vi "SignalSenderLoop.TestLauncher.vi"() -> ()   [LabVIEW 2020, in "ECU_Diagnose.lvlib" / "SignalSenderLoop.lvclass"]
doc: "JKI State Machine Objects (SMO) 1.0.0.5\nJKI - JKI\nCopyright (c) 2016, JKI"
uses:
  SignalSenderLoop.lvclass
  Typedefs/Data.ctl
  Typedefs/PublicEvents--Cluster.ctl
  Typedefs/SetpointChanged--EventData--Cluster.ctl
  <vilib>/JKI/JKI SMO/SMO/Typedefs/Public Events.ctl
  <vilib>/JKI/JKI SMO/SMO/Typedefs/SMOState --Enum.ctl
  <vilib>/JKI/JKI SMO/SMO/Typedefs/Reserve State--Enum.ctl
  <vilib>/JKI/JKI SMO/SMO/SMO.lvclass
  C:/Program Files (x86)/National Instruments/LabVIEW 2020/vi.lib/JKI/JKI SMO/SMO/SMO.lvclass
panel:
  out "SMOArry":refnum<class "SignalSenderLoop.lvclass">[](array[class])
  out "EventHandl(订阅事件用)":refnum<event-registration>[](array[refnum])
  in  "SignalsSet 2":dbl[](array[numeric])=[0.0]
  out "元素":refnum<class "SignalSenderLoop.lvclass">
  in  "SignalsSet":dbl[](array[numeric])=[60.0, 1.0]
  out "Value 3":T1
  out "Value 2":T1
  out "数组":errorcluster[](array[cluster])
  in  "Stop":bool
  # "ECU Signals Sender Test Launcher"
  # "数组为空，不发送任何帧，即停止发送"
  # "数组为空，不发送任何帧，即停止发送"
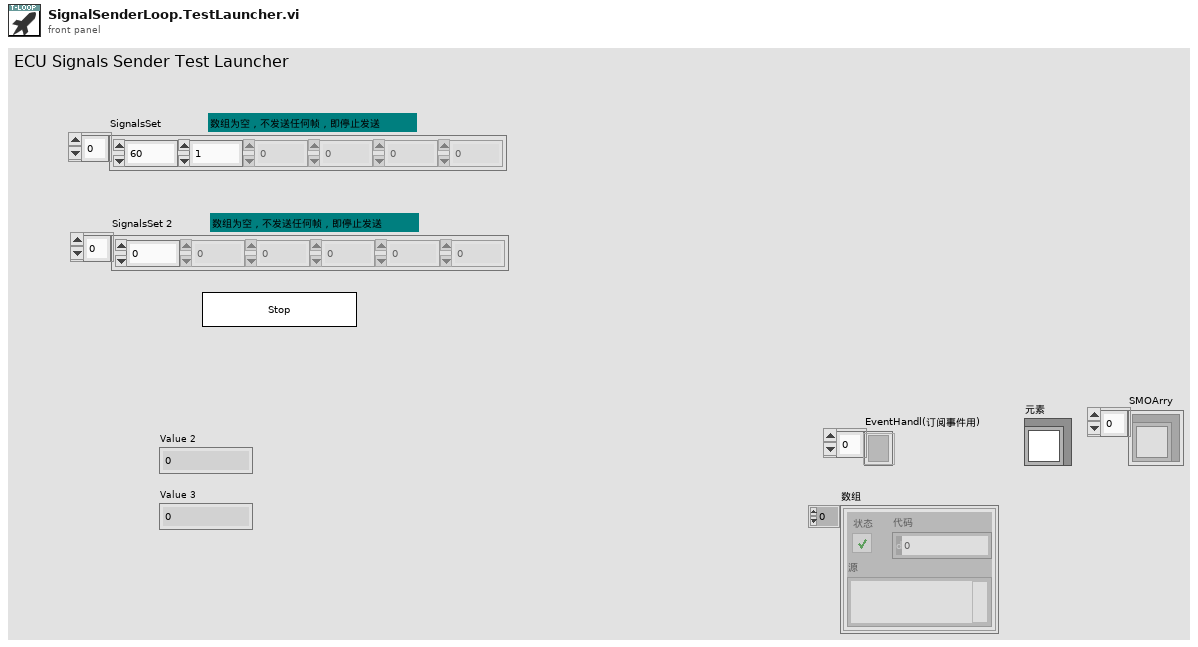
[diagram p1: front panel]
types:
  T1 = typedef "ECU_Diagnose.lvlib/SignalSenderLoop.lvclass/Data.ctl" = dbl
  T2 = typedef "SMO.lvclass/SMOState --Enum.ctl" = enum16{"unknown", "Created", "Started", "Stopped"}
  T3 = typedef "SignalSenderLoop.lvclass/Data.ctl" = dbl
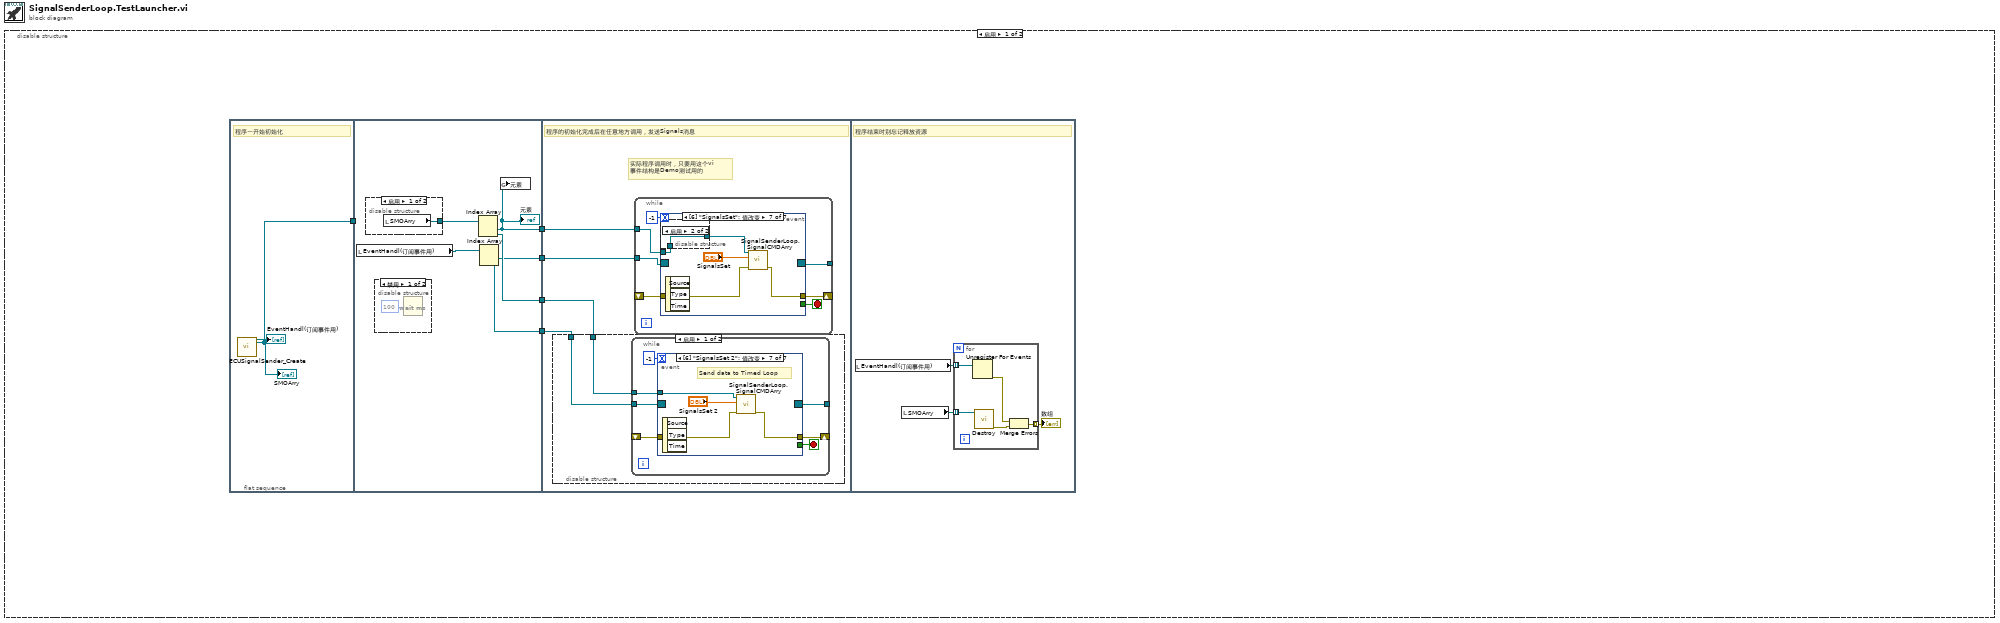
[diagram p0: block diagram]
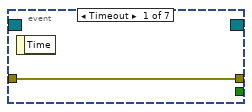
[diagram p4: hidden frame]
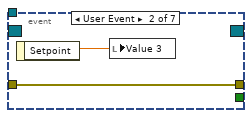
[diagram p5: hidden frame]
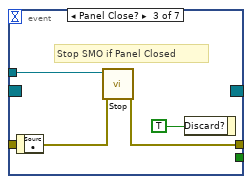
[diagram p6: hidden frame]
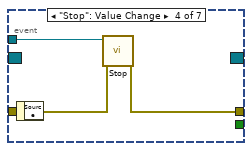
[diagram p7: hidden frame]
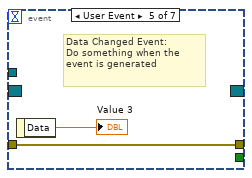
[diagram p8: hidden frame]
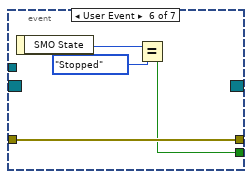
[diagram p9: hidden frame]
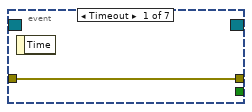
[diagram p11: hidden frame]
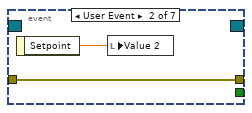
[diagram p12: hidden frame]
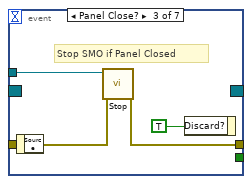
[diagram p13: hidden frame]
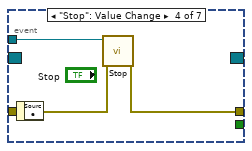
[diagram p14: hidden frame]
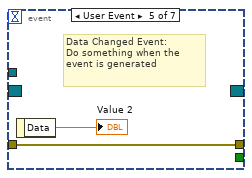
[diagram p15: hidden frame]
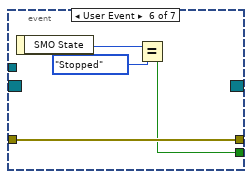
[diagram p16: hidden frame]
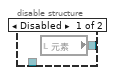
[diagram p17: hidden frame]
diagram:
  n1 = disable-structure shown="启用" {
    frame Enabled {
      n2 = flat-sequence {
        tunnel: [w6] -> w1
        tunnel: [w8] -> w5
        tunnel: [w11] -> w4
        tunnel: [w10] -> w3
        tunnel: [w9] -> w2
        tunnel: w1 -> [_]
        tunnel: w5 -> [w20]
        tunnel: w4 -> [w19]
        tunnel: w3 -> [w18]
        tunnel: w2 -> [w17]
        frame #0 {
          # "程序一开始初始化"
          n3 = call "ECUSignalSender_Create.vi"() -> ("EventHandl(订阅事件用)"=→"EventHandl(订阅事件用)":refnum<event-registration>[], "SMOArry"=w6:refnum<class "SignalSenderLoop.lvclass">[])  [unwired: 17 in, 1 out]
          "SMOArry" <- w6
        }
        frame #1 {
          n4 = local read "EventHandl(订阅事件用)"() -> (w12:refnum<event-registration>[])
          n5 = disable-structure shown="启用" {
            disable-tunnel: [w14 w15] -> w13
            frame Enabled {
              n6 = local read "SMOArry"() -> (w14:refnum<class "SignalSenderLoop.lvclass">[])
            }
            frame Disabled {
            }
          }
          n7 = disable-structure shown="禁用" {
            frame Disabled {
              n8 = Wait (ms)(milliseconds to wait=u32 100 ("等待时间（毫秒）")) -> ()  [unwired: 1 out]
            }
            frame Enabled {
            }
          }
          n9 = Index Array(array=w13) -> (element #1=w8:refnum<class "SignalSenderLoop.lvclass">, element #2=w11:refnum<class "SignalSenderLoop.lvclass">)  [unwired: 2 in]
          "元素" <- w8
          n10 = Index Array(array=w12) -> (element #1=w10:refnum<event-registration>, element #2=w9:refnum<event-registration>)  [unwired: 2 in]
          n11 = global write "test 1.vi" "元素"(w8) -> ()
        }
        frame #2 {
          # "实际程序调用时，只要用这个vi\n事件结构是Demo测试用的"
          # "程序的初始化完成后在任意地方调用，发送Signals消息"
          n12 = disable-structure shown="启用" {
            disable-tunnel: w17 -> [w22 _]
            disable-tunnel: w19 -> [w21 _]
            frame Enabled {
              n13 = while {
                shift-right: [w28] -> _
                shift-left: _ -> [w27]
                tunnel: w22 -> [w26]
                tunnel: [w25] -> _
                tunnel: w21 -> [w24]
                stop <- w29 stop-if-true
                n14 = event shown="[6] \"SignalsSet 2\": 值改变" {
                  selector: w26 -> [_ _ _ _ _ _ _]
                  dyn-events: [_ _ _ _ _ _ _] -> w25
                  timeout: -1 -> [_ _ _ _ _ _ _]
                  tunnel: [_ _ _ _ _ w42 _] -> w29
                  tunnel: w24 -> [_ _ w36 w39 _ _ w49]
                  tunnel: [w30 w32 w35 w38 w41 w45 w46] -> w28
                  tunnel: w27 -> [w30 w32 w34 w37 w41 w45 w47]
                  event Timeout {
                    n15 = event-data() -> ()  [unwired: 1 in, 1 out]
                  }
                  event User Event {
                    n16 = event-data() -> ("Setpoint"=w31:T3)  [unwired: 1 in]
                    n17 = local write "Value 3"(w31) -> ()
                  }
                  event Panel Close? {
                    # "Stop SMO if Panel Closed"
                    n18 = event-data() -> ()  [unwired: 1 in, 1 out]
                    n19 = call <vilib>:"Stop.vi"("error in (no error)"=w34, "SMO"=w36) -> ("error out"=w35:errorcluster)  [unwired: 8 in, 1 out]
                    n20 = event-data("Discard?"=TRUE ("OK")) -> ()  [unwired: 1 in, 1 out]
                  }
                  event "Stop": Value Change {
                    n21 = event-data() -> ()  [unwired: 1 in, 1 out]
                    n22 = call <vilib>:"Stop.vi"("error in (no error)"=w37, "SMO"=w39) -> ("error out"=w38:errorcluster)  [unwired: 8 in, 1 out]
                  }
                  event User Event {
                    # "Data Changed Event:\nDo something when the\nevent is generated"
                    n23 = event-data() -> ("Data"=→"Value 3":T3)  [unwired: 1 in]
                  }
                  event User Event {
                    n24 = event-data() -> ("SMO State"=w44:T2)  [unwired: 1 in]
                    n25 = Equal?(x=w44, y=SMOState_--Enum."Stopped") -> (x = y?=w42:bool)
                  }
                  event "SignalsSet 2": Value Change {
                    # "Send data to Timed Loop"
                    n26 = event-data() -> ()  [unwired: 1 in, 3 out]
                    n27 = call "SignalSenderLoop.SignalCMDArry.vi"("error in (no error)"=w47, "SignalCMDArry"="SignalsSet 2", "SignalSenderLoop"=w49) -> ("error out"=w46:errorcluster)  [unwired: 7 in, 1 out]
                  }
                }
              }
            }
            frame Disabled {
            }
          }
          n28 = while {
            shift-right: [w55] -> _
            shift-left: _ -> [w54]
            tunnel: [w53] -> _
            tunnel: w20 -> [w51]
            tunnel: w18 -> [w50]
            stop <- w56 stop-if-true
            n29 = event shown="[6] \"SignalsSet\": 值改变" {
              selector: w50 -> [_ _ _ _ _ _ _]
              dyn-events: [_ _ _ _ _ _ _] -> w53
              timeout: -1 -> [_ _ _ _ _ _ _]
              tunnel: [_ _ _ _ _ w69 _] -> w56
              tunnel: [w57 w59 w63 w66 w68 w72 w76] -> w55
              tunnel: w54 -> [w57 w59 w62 w65 w68 w72 w77]
              tunnel: w51 -> [_ _ w60 w64 _ _ w73]
              event Timeout {
                n30 = event-data() -> ()  [unwired: 1 in, 1 out]
              }
              event User Event {
                n31 = event-data() -> ("Setpoint"=w58:T3)  [unwired: 1 in]
                n32 = local write "Value 2"(w58) -> ()
              }
              event Panel Close? {
                # "Stop SMO if Panel Closed"
                n33 = event-data() -> ()  [unwired: 1 in, 1 out]
                n34 = call <vilib>:"Stop.vi"("error in (no error)"=w62, "SMO"=w60) -> ("error out"=w63:errorcluster)  [unwired: 8 in, 1 out]
                n35 = event-data("Discard?"=TRUE ("OK")) -> ()  [unwired: 1 in, 1 out]
              }
              event "Stop": Value Change {
                n36 = event-data() -> ()  [unwired: 1 in, 1 out]
                n37 = call <vilib>:"Stop.vi"("error in (no error)"=w65, "SMO"=w64) -> ("error out"=w66:errorcluster)  [unwired: 8 in, 1 out]
              }
              event User Event {
                # "Data Changed Event:\nDo something when the\nevent is generated"
                n38 = event-data() -> ("Data"=→"Value 2":T3)  [unwired: 1 in]
              }
              event User Event {
                n39 = event-data() -> ("SMO State"=w71:T2)  [unwired: 1 in]
                n40 = Equal?(x=w71, y=SMOState_--Enum."Stopped") -> (x = y?=w69:bool)
              }
              event "SignalsSet": Value Change {
                n41 = disable-structure shown="启用" {
                  disable-tunnel: [w78 w79] -> w74
                  disable-tunnel: w73 -> [_ w79]
                  frame Disabled {
                    n42 = local read "元素"() -> (w78:refnum<class "SignalSenderLoop.lvclass">)
                  }
                  frame Enabled {
                  }
                }
                n43 = event-data() -> ()  [unwired: 1 in, 3 out]
                n44 = call "SignalSenderLoop.SignalCMDArry.vi"("error in (no error)"=w77, "SignalCMDArry"="SignalsSet", "SignalSenderLoop"=w74) -> ("error out"=w76:errorcluster)  [unwired: 7 in, 1 out]
              }
            }
          }
        }
        frame #3 {
          # "程序结束时别忘记释放资源"
          n45 = local read "EventHandl(订阅事件用)"() -> (w81:refnum<event-registration>[])
          n46 = local read "SMOArry"() -> (w80:refnum<class "SignalSenderLoop.lvclass">[])
          n47 = for {
            tunnel: w81 -> [w87] mode=indexing
            tunnel: [w84] -> w82 mode=indexing
            tunnel: w80 -> [w83] mode=indexing
            n48 = Unregister For Events(event registration refnum=w87) -> (error out=w86:errorcluster)  [unwired: 1 in]
            n49 = call <vilib>:"Destroy.vi"("SMO"=w83) -> ("error out"=w85:errorcluster)  [unwired: 10 in]
            n50 = Merge Errors(w86, w85) -> (w84:errorcluster)
          }
          "数组" <- w82
        }
      }
    }
    frame Disabled {
    }
  }
